vi "Test Process Cleared on Upstream Error.vi"(8 "error in (no error)":errorcluster, 11 "Process Test In":refnum<class "Process Test.lvclass">) -> (0 "error out":errorcluster, 3 "Process Test Out":refnum<class "Process Test.lvclass">)   [LabVIEW 2020, in "Process Test.lvclass"]
uses:
  Process Test.lvclass
  C:/Users/anton/Documents/GitHub/Triarc-Framework/source/Framework Test/Base Class Test/Base Test.lvclass
  C:/Program Files (x86)/National Instruments/LabVIEW 2020/vi.lib/Asteme/LUnit/Test Case.lvclass
  Framework/Process/Process.lvclass
  Framework/Process/Public/Lifecycle/Lifecycle State.ctl
  Base Class Test/Base Test.lvclass/Base Test.ctl
  Framework/Process/Process.lvclass/Process.ctl
  <vilib>/Asteme/LUnit/Test Case.lvclass/Test Case.ctl
  <vilib>/Asteme/LUnit/LUnit Assertion Result.lvclass/LUnit Assertion Result.ctl
  <vilib>/Asteme/LUnit/Palette/Fail.vi
  <vilib>/Asteme/LUnit/Palette/Pass.vi
  <vilib>/Asteme/LUnit/Set Assertion Type.vi
  <vilib>/Asteme/LUnit/Add test result.vi
  <vilib>/Asteme/LUnit/LUnit Write Passed.vi
  <vilib>/Asteme/LUnit/LUnit Get Test Case.vi
  <vilib>/Asteme/LUnit/Assertion Result/LUnit Get Test Name.vi
  <vilib>/Asteme/LUnit/LUnit Write Message.vi
  <vilib>/Asteme/LUnit/LUnit Write Description.vi
  <vilib>/Asteme/LUnit/LUnit Write Assertion Type.vi
  <vilib>/Asteme/LUnit/Read Test Case Name.vi
  Framework/Base/Base.lvclass
  <vilib>/Asteme/LUnit/LUnit Assertion Result.lvclass
  Base Class Test/Base Test.lvclass
  <vilib>/Asteme/LUnit/Test Case.lvclass
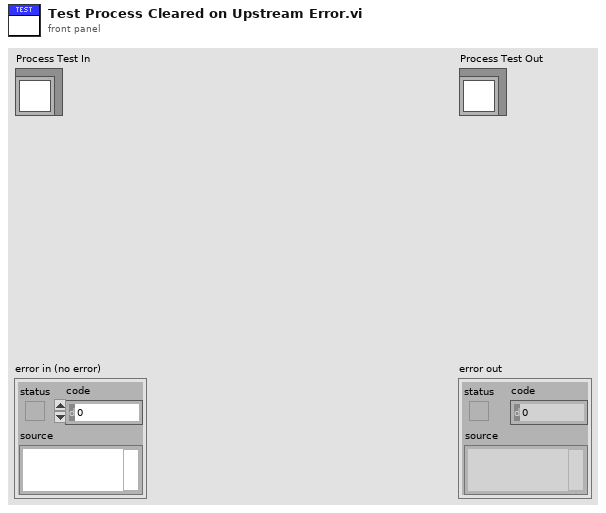
[diagram p1: front panel]
types:
  T1 = typedef "Process.lvclass/Lifecycle State.ctl" = enum16{"Uninitialized", "Initialized", "Started", "Running", "Stopped", "Finished"}
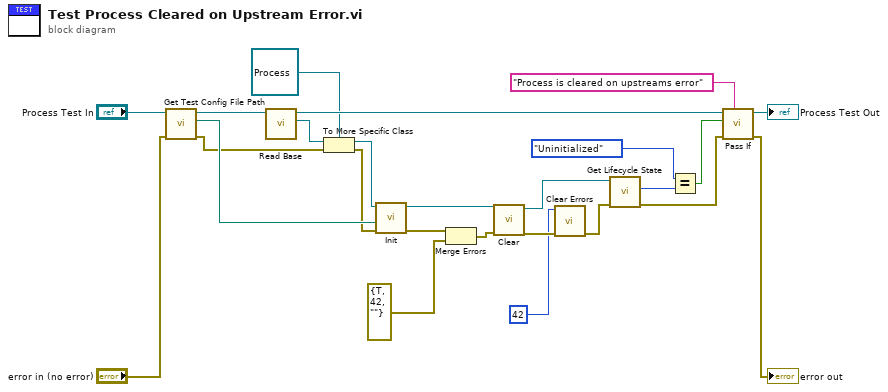
[diagram p0: block diagram]
diagram:
  n1 = call-dynamic "Get Test Config File Path.vi"("error in (no error)"="error in (no error)", "Base Class Test in"="Process Test In") -> ("error out"=w14:errorcluster, "Test config path"=w20:path, "Base Class Test out"=w22:refnum<class "Process Test.lvclass">)  [unwired: 7 in]
  n2 = call "Read Base.vi"("Base Class Test In"=w22) -> ("Base.lvclass"=w17:refnum<class "Base.lvclass">, "Base Class Test Out"=w19:refnum<class "Process Test.lvclass">)  [unwired: 8 in, 1 out]
  n3 = To More Specific Class(target class=refnum<class "Process.lvclass"> refnum ("Process.lvclass"), reference=w17, error in=w14) -> (specific class reference=w16:refnum<class "Process.lvclass">, error out=w15:errorcluster)
  n4 = call-dynamic "Init.vi"("error in (no error)"=w15, "Config File Path"=w20, "Process In"=w16) -> ("error out"=w23:errorcluster, "Process Out"=w24:refnum<class "Process.lvclass">)  [unwired: 7 in]
  n5 = Merge Errors(w23, errorcluster {"status"=TRUE, "code"=42, "source"=""} ("error constant")) -> (w2:errorcluster)
  n6 = call-dynamic "Clear.vi"("error in (no error)"=w2, "Process In"=w24) -> ("error out"=w6:errorcluster, "Process Out"=w13:refnum<class "Process.lvclass">)  [unwired: 8 in]
  n7 = call <vilib>:"Clear Errors.vi"("error in (no error)"=w6, "specific error code to clear (0: all)"=42 ("code")) -> ("error out"=w5:errorcluster)  [unwired: 4 in, 1 out]
  n8 = call "Get Lifecycle State.vi"("error in (no error)"=w5, "Process In"=w13) -> ("error out"=w8:errorcluster, "Lifecycle State"=w10:T1)  [unwired: 6 in, 2 out]
  n9 = Equal?(x=Lifecycle_State."Uninitialized" ("Lifecycle State"), y=w10) -> (x = y?=w9:bool)
  n10 = call <vilib>:"Pass If.vi"("Description"="Process is cleared on upstreams error", "error in (no error)"=w8, "Pass?"=w9, "Test Case In"=w19) -> ("error out"=→"error out":errorcluster, "Test Case Out"=→"Process Test Out":refnum<class "Process Test.lvclass">)  [unwired: 6 in]
